vi "Set Wheel Parameter by Name.vi"(8 "error in (no error)":errorcluster, 9 "parameter value":variant, 10 "parameter name":string, 11 "wheel in":refnum<class "NI_Robotics_Mecanum Wheel.lvclass">) -> (0 "error out":errorcluster, 1 "set?":bool, 3 "wheel out":refnum<class "NI_Robotics_Mecanum Wheel.lvclass">)   [LabVIEW 2017, in "NI_Robotics_Mecanum Wheel.lvclass"]
uses:
  <vilib>/robotics/Steering/Mecanum Wheel/NI_Robotics_Mecanum Wheel.lvclass
  <vilib>/robotics/Steering/Mecanum Wheel/Roller Orientation.ctl
  <vilib>/robotics/Steering/Mecanum Wheel/NI_Robotics_Mecanum Wheel.lvclass/NI_Robotics_Mecanum Wheel.ctl
  <vilib>/robotics/Steering/Wheel/NI_Robotics_Wheel.lvclass
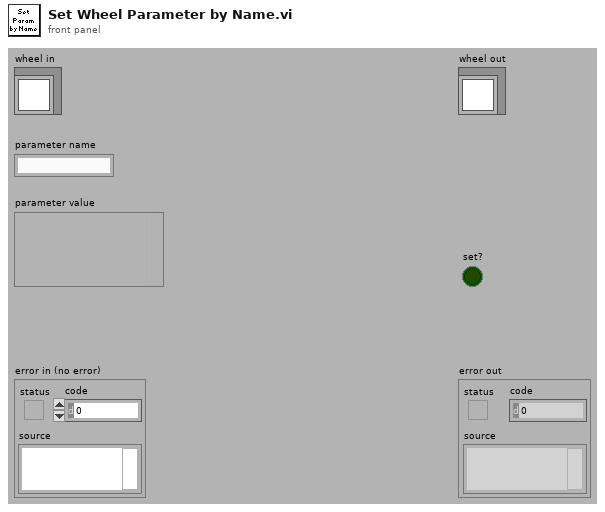
[diagram p1: front panel]
types:
  T1 = typedef "NI_Robotics_Mecanum Wheel.lvclass/Roller Orientation.ctl" = u16
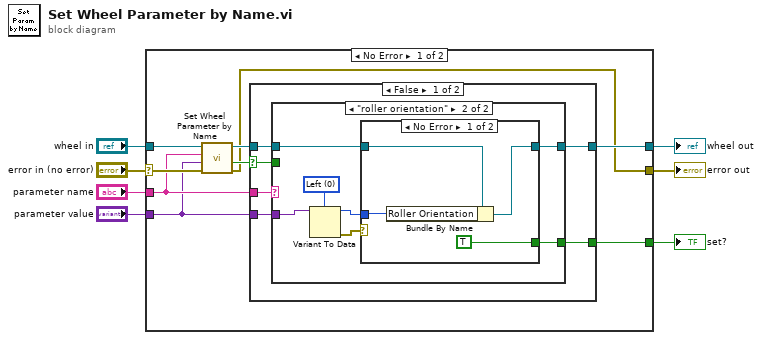
[diagram p0: block diagram]
diagram:
  n1 = case shown="No Error" "error in (no error)" {
    selector: "error in (no error)" -> [w15 w38]
    tunnel: "parameter value" -> [w9 _]
    tunnel: "parameter name" -> [w10 _]
    tunnel: "wheel in" -> [w16 w39]
    tunnel: [w12 w39] -> w3
    tunnel: [w11 _] -> w2
    tunnel: [w8 w38] -> w1
    frame No Error {
      n2 = call-parent "Set Wheel Parameter by Name.vi"("error in (no error)"=w15, "parameter value"=w9, "parameter name"=w10, "wheel in"=w16) -> ("error out"=w8:errorcluster, "set?"=w13:bool, "wheel out"=w14:refnum<class "NI_Robotics_Mecanum Wheel.lvclass">)  [unwired: 5 in]
      n3 = case shown="False" w13 {
        selector: w13 -> [w19 w36]
        tunnel: w14 -> [w22 w37]
        tunnel: [w20 w37] -> w12
        tunnel: w10 -> [w21 _]
        tunnel: [w18 w36] -> w11
        tunnel: w9 -> [w17 _]
        frame False {
          n4 = case shown="\"roller orientation\"" w21 {
            tunnel: w22 -> [w23 w30]
            tunnel: [w23 w29] -> w20
            tunnel: w19 -> [_ _]
            tunnel: [_ w25] -> w18
            tunnel: w17 -> [_ w28]
            frame Default {
            }
            frame "roller orientation" {
              w24 = T1 0 items=["Left", "Right"] ("Roller Orientation")
              n5 = Variant To Data(type=w24, Variant=w28) -> (data=w26:T1, error out=w27:errorcluster)  [unwired: 1 in]
              n6 = case shown="No Error" w27 {
                tunnel: w30 -> [w34 w35]
                tunnel: [w33 w35] -> w29
                tunnel: w26 -> [w31 _]
                tunnel: [TRUE _] -> w25
                frame No Error {
                  n7 = Bundle By Name(cluster=w34, "Roller Orientation"=w31) -> (w33:refnum<class "NI_Robotics_Mecanum Wheel.lvclass">)
                }
                frame Error {
                }
              }
            }
          }
        }
        frame True {
        }
      }
    }
    frame Error {
    }
  }
  "error out" <- w1
  "wheel out" <- w3
  "set?" <- w2
